vi "RudderToPoint.vi"(1 "Angle to Check":dbl) -> (8 "Goodness":dbl)   [LabVIEW 2012]
doc: "Takes in an angle to check, and returns a goodness value related to how close said angle is to the angle between the robot and the waypoint.\n\nTODO: Convert to using angle class"
uses:
  Data/TypeDefs/UTM Location.ctl
  Utilities/Math/Angles/Angle/Angle.lvclass
panel:
  in  "Robot Angle":dbl
  in  "Robot Location":T1 {"North" format="%#_10f"; "East" format="%#_8f"}
  in  "Waypoint":T1 {"North" format="%#_10f"; "East" format="%#_8f"}
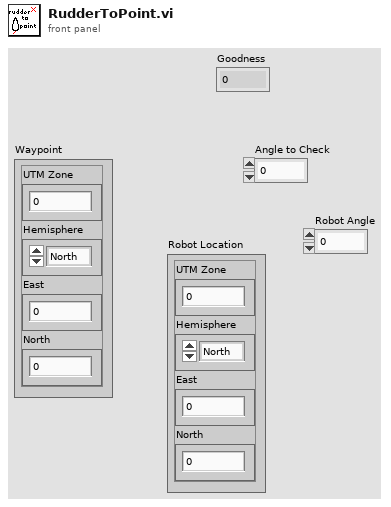
[diagram p1: front panel]
types:
  T1 = typedef "UTM Location.ctl" = cluster{"UTM Zone":dbl, "Hemisphere":enum16{"North", "South"}, "East":dbl, "North":dbl}
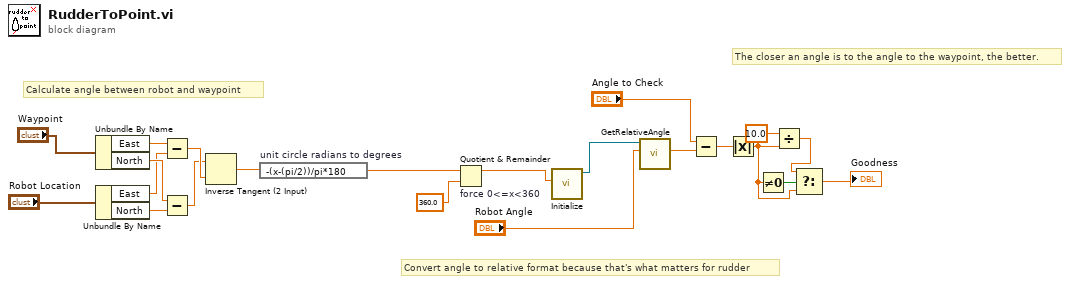
[diagram p0: block diagram]
diagram:
  # "The closer an angle is to the angle to the waypoint, the better."
  # "Convert angle to relative format because that's what matters for rudder"
  # "Calculate angle between robot and waypoint"
  n1 = Unbundle By Name("Waypoint") -> ("East"=w17:dbl, "North"=w19:dbl)
  n2 = Unbundle By Name("Robot Location") -> ("East"=w18:dbl, "North"=w20:dbl)
  n3 = Subtract(x=w17, y=w18) -> (x-y=w22:dbl)
  n4 = Subtract(x=w19, y=w20) -> (x-y=w21:dbl)
  n5 = Inverse Tangent (2 Input) ("use inverse tangent\nto get heading")(1:w22, 2:w21) -> (0:w12:dbl)
  n6 = expression code="-(x-(pi/2))/pi*180" "unit circle radians to degrees"(w12) -> (w13:dbl)
  n7 = Quotient & Remainder "force 0<=x<360"(x=w13, y=360.0) -> (x-y*floor(x/y)=w11:dbl)  [unwired: 1 out]
  n8 = call "Initialize.vi"("Input Angle (Deg.)"=w11) -> ("Angle out"=w10:refnum<class "Angle.lvclass">)  [unwired: 9 in, 1 out]
  n9 = call "GetRelativeAngle.vi"("Boat Angle (Deg.)"="Robot Angle", "Angle in"=w10) -> ("Relative Angle"=w8:dbl)  [unwired: 8 in, 1 out]
  n10 = Subtract(x="Angle to Check", y=w8) -> (x-y=w6:dbl)
  n11 = Absolute Value(x=w6) -> (abs(x)=w2:dbl)
  n12 = Not Equal To 0?(x=w2) -> (x != 0?=w4:bool)
  n13 = Divide(x=10.0, y=w2) -> (x/y=w3:dbl)
  n14 = Select(t=w3, s=w4, f=w2) -> (s? t:f=→"Goodness":dbl)
